vi "Filter Example 3 channel.vi"() -> ()   [LabVIEW 2009]
uses:
  <vilib>/ptbypt/NI_PtbyPt.lvlib
panel:
  out "Channel 3":dbl(knob)=0.823298640430447 scale=0.0..1.0
  out "Chan 3":dbl=0.823298640430447
  out "Channel 2":dbl(knob)=0.9540153437529694 scale=0.0..1.0
  out "Chan 2":dbl=0.9540153437529694
  out "Chan 1":dbl=0.165419862799715
  out "Channel 1":dbl(knob)=0.165419862799715 scale=0.0..1.0
  in  "stop":bool
  in  "print 4":bool
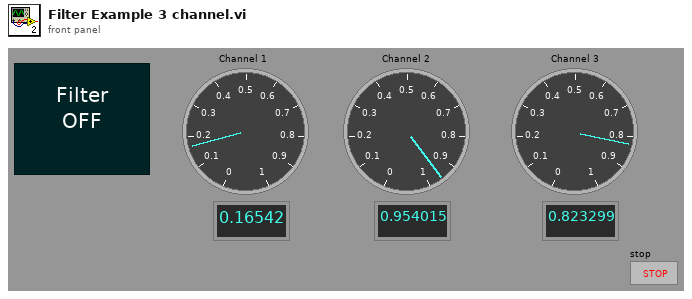
[diagram p1: front panel]
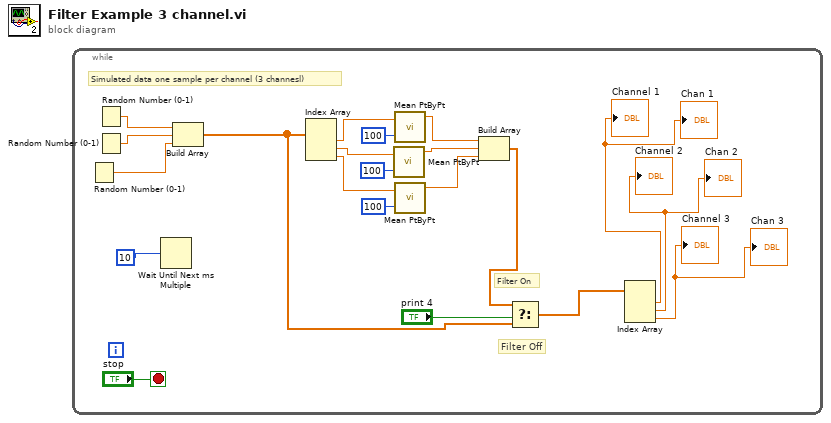
[diagram p0: block diagram]
diagram:
  n1 = while {
    stop <- "stop" stop-if-true
    # "Filter Off"
    # "Filter On"
    # "Simulated data one sample per channel (3 channesl)"
    n2 = Random Number (0-1)() -> (number: 0 to 1=w8:dbl)
    n3 = Random Number (0-1)() -> (number: 0 to 1=w6:dbl)
    n4 = Random Number (0-1)() -> (number: 0 to 1=w7:dbl)
    n5 = Wait Until Next ms Multiple(millisecond multiple=10) -> ()  [unwired: 1 out]
    n6 = Build Array(w6, w7, w8) -> (w5:dbl[])
    n7 = Index Array(array=w5) -> (element #1=w17:dbl, element #2=w18:dbl, element #3=w19:dbl)  [unwired: 3 in]
    n8 = call <vilib>:"Mean PtByPt.vi"("x"=w18, "sample length"=100) -> ("mean"=w12:dbl)  [unwired: 1 in, 2 out]
    n9 = call <vilib>:"Mean PtByPt.vi"("x"=w17, "sample length"=100) -> ("mean"=w13:dbl)  [unwired: 1 in, 2 out]
    n10 = call <vilib>:"Mean PtByPt.vi"("x"=w19, "sample length"=100) -> ("mean"=w11:dbl)  [unwired: 1 in, 2 out]
    n11 = Build Array(w13, w12, w11) -> (w10:dbl[])
    n12 = Select(t=w10, s="print 4", f=w5) -> (s? t:f=w4:dbl[])
    n13 = Index Array(array=w4) -> (element #1=→"Channel 1" →"Chan 1":dbl, element #2=→"Channel 2" →"Chan 2":dbl, element #3=→"Channel 3" →"Chan 3":dbl)  [unwired: 3 in]
  }
